vi "LogotipoUPIITAHDFinal.vi"() -> ()   [LabVIEW 2016]
uses:
  <vilib>/DAQmx/write.llb/DAQmx Write (Analog 2D DBL NChan NSamp).vi
  <vilib>/DAQmx/create/channels.llb/DAQmx Create Channel (AO-Voltage-Basic).vi
  <vilib>/DAQmx/configure/timing.llb/DAQmx Timing (Sample Clock).vi
  <vilib>/DAQmx/miscellaneous.llb/DAQmx Fill In Error Info.vi
panel:
  in  "Stop Button":bool
  out "X":dbl[](graph)
  out "Y":dbl[](graph)
  out "XY Graph":cluster{dbl[], dbl[]}(graph)
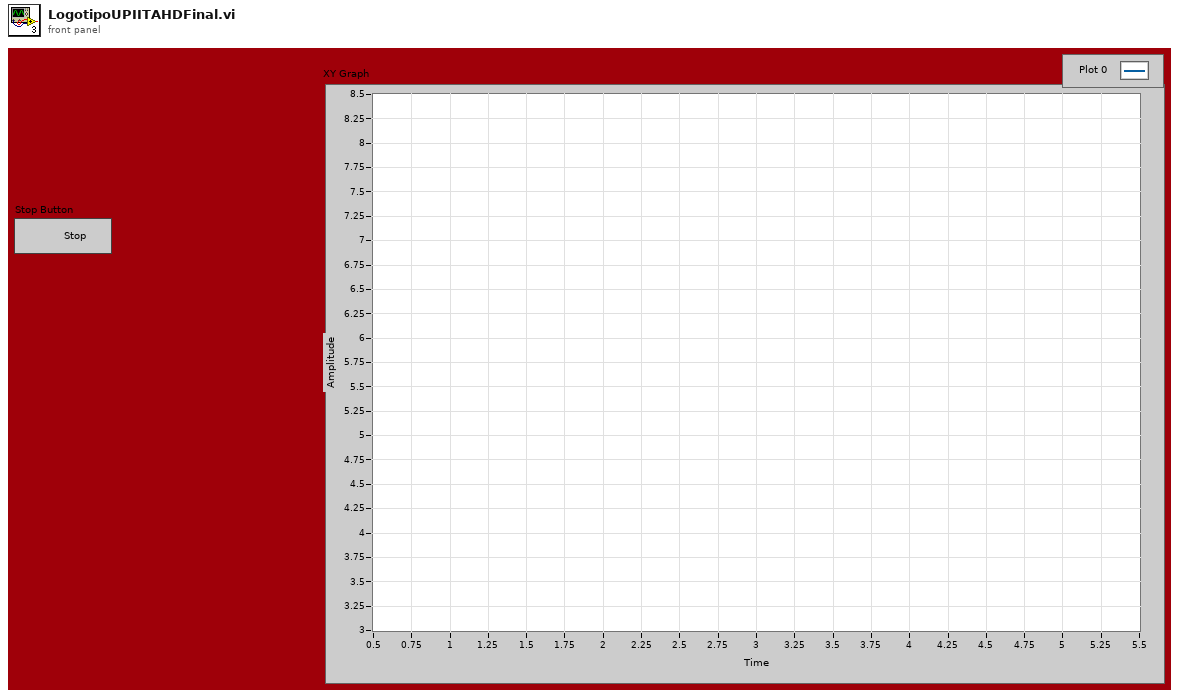
[diagram p1: front panel]
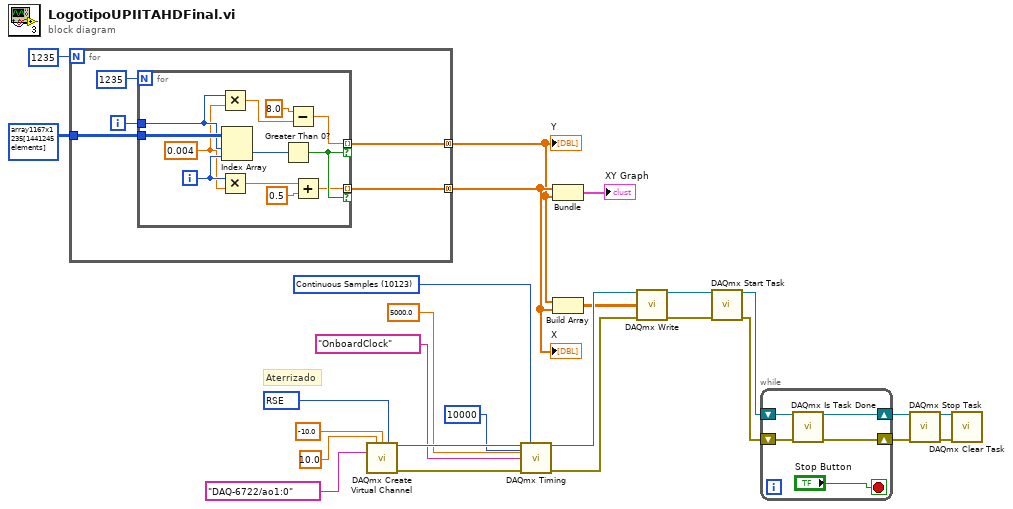
[diagram p0: block diagram]
diagram:
  w1 = 10123 items=["Finite Samples"=10178, "Continuous Samples"=10123, "Hardware Timed Single Point"=12522] ("sample mode")
  w19 = 10083 items=["Default"=-1, "RSE"=10083, "NRSE"=10078, "Differential"=10106, "Pseudodifferential"=12529] ("input terminal configuration")
  # "Aterrizado"
  n1 = for {
    N: 1235 -> [_]
    tunnel: i16[][] array1167x1235[1441245 elements] ("IMAGEN") -> [w31]
    tunnel: [w27] -> w23 mode=concatenating
    tunnel: [w28] -> w24 mode=concatenating
    i -> [w30]
    n2 = for {
      N: 1235 -> [_]
      tunnel: w31 -> [w43]
      tunnel: w30 -> [w39]
      tunnel: [w32] -> w28 mode=indexing if=w41
      tunnel: [w35] -> w27 mode=indexing if=w41
      i -> [w40]
      w38 = 0.004 ("y")
      n3 = Multiply(x=w39, y=w38) -> (x*y=w36:dbl)
      n4 = Multiply(x=w40, y=w38) -> (x*y=w34:dbl)
      n5 = Index Array(array=w43, index (row)=w39, index (col)=w40) -> (element=w42:i16)
      n6 = Greater Than 0?(x=w42) -> (x > 0?=w41:bool)
      n7 = Subtract(x=8.0 ("y"), y=w36) -> (x-y=w35:dbl)
      n8 = Add(x=w34, y=0.5) -> (x+y=w32:dbl)
    }
  }
  "Y" <- w23
  "X" <- w24
  n9 = call-poly <vilib>:"DAQmx Create Virtual Channel.vi"("maximum value"=10.0, "minimum value"=-10.0, "output terminal configuration"=w19, "physical channels"=tag "DAQ-6722/ao1:0") -> ("task out"=w15:refnum<k21>, "error out"=w14:errorcluster)  [unwired: 10 in]
  n10 = call-poly <vilib>:"DAQmx Timing.vi"("task/channels in"=w15, "sample mode"=w1, "samples per channel"=10000, "rate"=5000.0, "source"=tag "OnboardClock", "error in"=w14) -> ("task out"=w10:refnum<k21>, "error out"=w9:errorcluster)  [unwired: 8 in]
  n11 = Bundle(w24, w23) -> (→"XY Graph":cluster{dbl[], dbl[]})  [unwired: 1 in]
  n12 = Build Array(w23, w24) -> (w2:dbl[][])
  n13 = call-poly <vilib>:"DAQmx Write.vi"("task/channels in"=w10, "data"=w2, "error in"=w9) -> ("task out"=w8:refnum<k21>, "error out"=w7:errorcluster)  [unwired: 10 in, 1 out]
  n14 = call <vilib>:"DAQmx Start Task.vi"("task/channels in"=w8, "error in"=w7) -> ("task out"=w6:refnum<k21>, "error out"=w5:errorcluster)  [unwired: 12 in]
  n15 = while {
    shift-right: [w46] -> w4
    shift-left: w6 -> [w48]
    shift-right: [w45] -> w3
    shift-left: w5 -> [w47]
    stop <- "Stop Button" stop-if-true
    n16 = call <vilib>:"DAQmx Is Task Done.vi"("task/channels in"=w48, "error in"=w47) -> ("task out"=w46:refnum<k21>, "error out"=w45:errorcluster)  [unwired: 11 in, 1 out]
  }
  n17 = call <vilib>:"DAQmx Stop Task.vi"("task/channels in"=w4, "error in"=w3) -> ("task out"=w18:refnum<k21>, "error out"=w17:errorcluster)  [unwired: 12 in]
  n18 = call <vilib>:"DAQmx Clear Task.vi"("task in"=w18, "error in"=w17) -> ()  [unwired: 13 in, 1 out]
